vi "subDFD_Get Control Value by Name.vi"(8 "error IO":errorcluster, 9 "Control Name":string, 11 "vi reference in":refnum<vi>) -> (0 "error out":errorcluster, 1 "Value":variant, 3 "vi reference out":refnum<vi>)   [LabVIEW 2023]
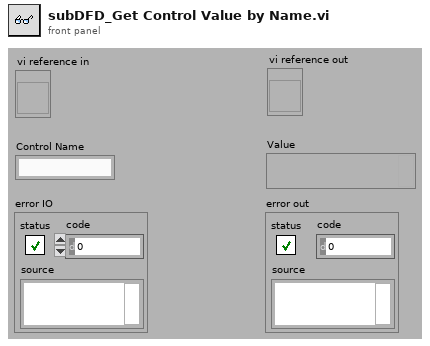
[diagram p1: front panel]
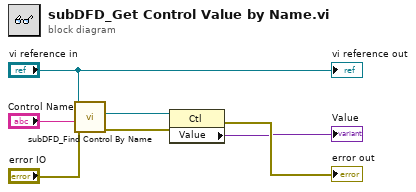
[diagram p0: block diagram]
diagram:
  n1 = call <vilib>:"subDFD_Find Control By Name.vi"("error in (no error)"="error IO", "control name"="Control Name", "vi refnum in"="vi reference in") -> ("error out"=w2:errorcluster, "control refnum"=w7:refnum<vi>)  [unwired: 1 in, 6 out]
  n2 = property class="Ctl"(reference=w7, error in=w2) -> (error out=→"error out":errorcluster, "Value"=→"Value":variant)  [unwired: 1 out]
  "vi reference out" <- "vi reference in"
